vi "getCurrentPosition.vi"(0 "reference (in)":refnum<class "_SingleAxisController.lvclass">, 2 "nc (single axis controllers require no axis specification)":T1, 5 "error in (no error)":errorcluster) -> (14 "reference (out)":refnum<class "_SingleAxisController.lvclass">, 16 "current_position (units)":i32, 19 "error out":errorcluster)   [LabVIEW 2020, in "classes.lvlib" / "_SingleAxisController.lvclass"]
doc: "Produced By:\n\n<B>Kod Integrations, LLC</B>\n4835 Marianne Drive\nMount Airy, MD 21771\nhttp://www.kodintegrations.com\nemail: info@kodintegrations.com\nphone: (240) 687-1288"
uses:
  _SingleAxisController.lvclass
  C:/GEECS/Developers Version/source/Device Drivers/Newmark-NSC-A/Arcus Driver 3.0.0/ArcusUsbComm/classes/Controller/_Controller.lvclass
  common/controls/axis.ctl
  Controller/_Controller.lvclass
  libraries/common.lvlib
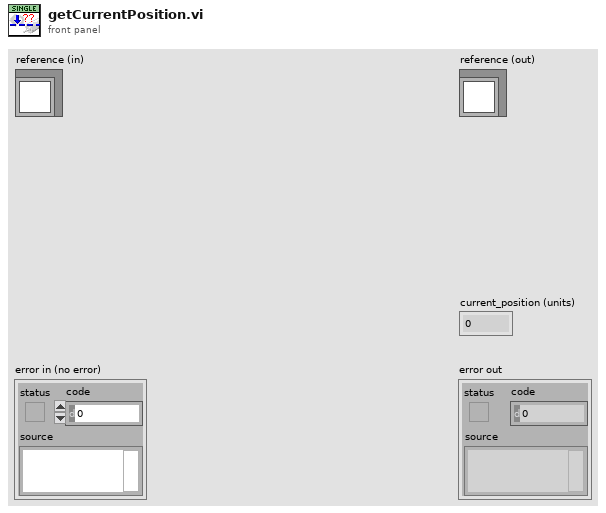
[diagram p1: front panel]
types:
  T1 = typedef "common.lvlib/axis.ctl" = enum16{"X", "Y", "Z", "U"}
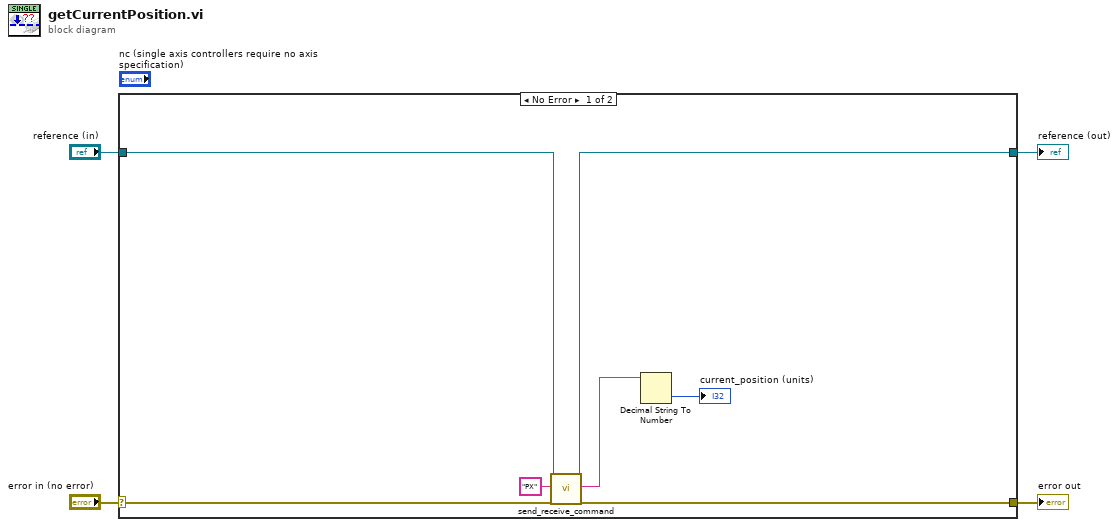
[diagram p0: block diagram]
diagram:
  n1 = case shown="No Error" "error in (no error)" {
    selector: "error in (no error)" -> [w9 w13]
    tunnel: [w8 w13] -> w3
    tunnel: [w10 w12] -> w1
    tunnel: "reference (in)" -> [w11 w12]
    frame No Error {
      n2 = call "send_receive_command.vi"("reference (in)"=w11, "ASCII Command (in)"="PX", "error in (no error)"=w9) -> ("reference (out)"=w10:refnum<class "_SingleAxisController.lvclass">, "response (out)"=w5:string, "error out"=w8:errorcluster)  [unwired: 12 in, 2 out]
      n3 = Decimal String To Number(string=w5) -> (number=→"current_position (units)":i32)  [unwired: 2 in, 1 out]
    }
    frame Error {
    }
  }
  "error out" <- w3
  "reference (out)" <- w1
